vi "Nonlinear Curve Fit LM formula string.vi"(0 "Y":dbl[](array[numeric]), 1 "initial parameters":dbl[](array[numeric]), 5 "X":dbl[](array[numeric]), 7 "Weight":dbl[](array[numeric]), 9 "model description":T2, 11 "error in (no error)":errorcluster, 12 "termination":cluster{"max iteration":i32, "tolerance":dbl}={"max iteration"=200, "tolerance"=1e-08}) -> (4 "best nonlinear fit":dbl[](array[numeric]), 6 "best fit parameters":dbl[](array[numeric]), 8 "covariance":T1, 14 "residue":dbl, 15 "error out":errorcluster)   [LabVIEW 2020, in "NI_Gmath.lvlib"]
doc: "Uses the Levenberg-Marquardt algorithm to determine the set of parameters that best fit the set of input data points (<B>X</B>, <B>Y</B>) as expressed by a nonlinear function y = <B>f(x,a)</B>, where a is the set of parameters. You must manually select the polymorphic instance to use."
uses:
  <vilib>/gmath/NI_Gmath.lvlib
  <vilib>/Analysis/Matrix/Datatypes/RealMatrix.ctl
  <vilib>/Analysis/Matrix/NI_Matrix.lvlib
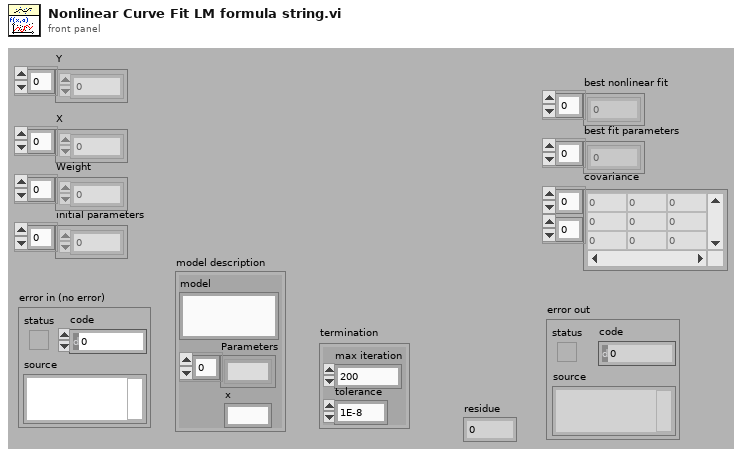
[diagram p1: front panel]
types:
  T1 = typedef "NI_Matrix.lvlib/RealMatrix.ctl" = dbl[][]
  T2 = cluster{"model":string, "Parameters":string[], "x":string}
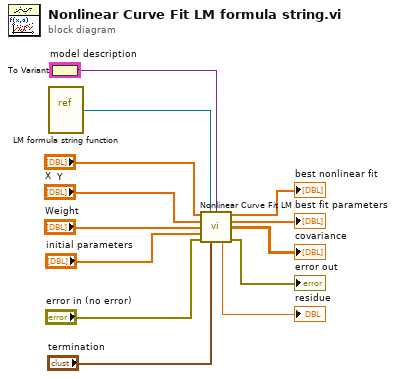
[diagram p0: block diagram]
diagram:
  n1 = vi-ref <vilib>:"LM formula string function.vi"() -> ("vi reference"=w2:refnum<vi>)
  n2 = To Variant(anything="model description") -> (Variant=w1:variant)
  n3 = call <vilib>:"Nonlinear Curve Fit LM.vi"("Y"="Y", "f(x,a)"=w2, "data"=w1, "X"="X", "Weight"="Weight", "initial parameters"="initial parameters", "error in (no error)"="error in (no error)", "termination"="termination") -> ("best nonlinear fit"=→"best nonlinear fit":dbl[], "best fit parameters"=→"best fit parameters":dbl[], "covariance"=→"covariance":T1, "residue"=→"residue":dbl, "error out"=→"error out":errorcluster)  [unwired: 2 in, 1 out]
